vi "Initialize.vi"(8 "error in (no error)":errorcluster, 11 "object in":refnum<class "NXP.lvclass">) -> (0 "error out":errorcluster, 3 "object out":refnum<class "NXP.lvclass">)   [LabVIEW 2020, in "NXP.lvclass"]
uses:
  NXP.lvclass
  Abstract/Serial Device/Serial Device.lvclass
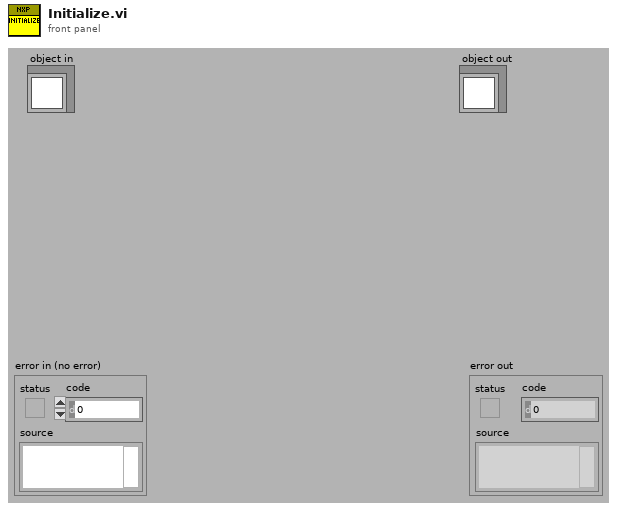
[diagram p1: front panel]
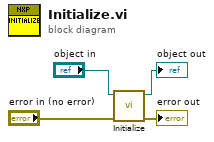
[diagram p0: block diagram]
diagram:
  n1 = call-parent "Initialize.vi"("error in (no error)"="error in (no error)", "object in"="object in") -> ("error out"=→"error out":errorcluster, "object out"=→"object out":refnum<class "NXP.lvclass">)  [unwired: 8 in]
